vi "Read IP address.vi"(8 "error in (no error)":errorcluster, 11 "Modbus Slave configuration in":refnum<class "Modbus Module configuration.lvclass">) -> (0 "error out":errorcluster, 2 "IP address":string, 3 "Modbus Slave configuration out":refnum<class "Modbus Module configuration.lvclass">)   [LabVIEW 2013, in "Modbus Module configuration.lvclass"]
uses:
  Modbus Module configuration.lvclass
  Modbus Module configuration.lvclass/Modbus Module configuration.ctl
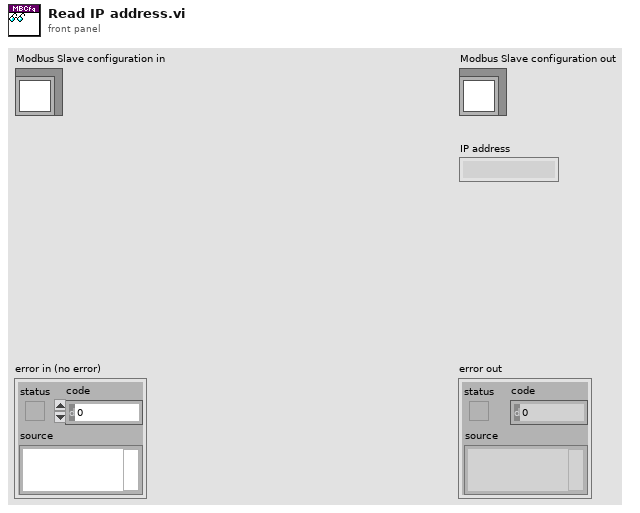
[diagram p1: front panel]
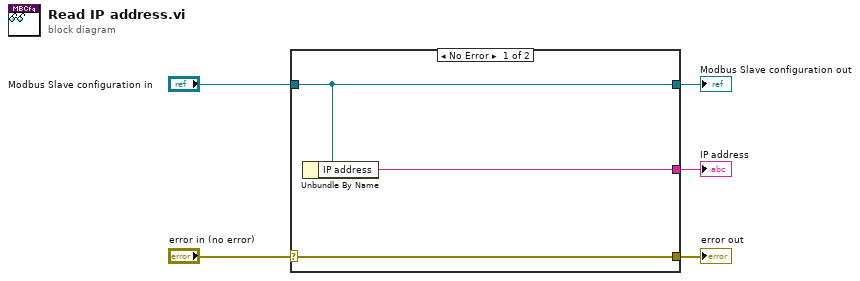
[diagram p0: block diagram]
diagram:
  n1 = case shown="No Error" "error in (no error)" {
    selector: "error in (no error)" -> [w8 w9]
    tunnel: [w8 w9] -> w4
    tunnel: [w7 w10] -> w2
    tunnel: "Modbus Slave configuration in" -> [w7 w10]
    tunnel: [w6 _] -> w1
    frame No Error {
      n2 = Unbundle By Name(w7) -> ("IP address"=w6:string)
    }
    frame Error {
    }
  }
  "error out" <- w4
  "Modbus Slave configuration out" <- w2
  "IP address" <- w1
